vi "Module Not Synced--error.vi"() -> (0 "error out":errorcluster)   [LabVIEW 2020, in "TCP Client.lvlib"]
doc: "Outputs an error cluster containing a custom error code indicating the module events were unable to synchronize.\n_____\nBased on DQMH Project Template 6.0.0.91."
uses:
  TCP Client.lvlib
  <vilib>/Utility/error.llb/Error Cluster From Error Code.vi
  <vilib>/ErrorRing/Error Ring.xnode
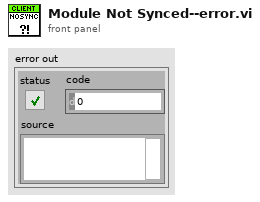
[diagram p1: front panel]
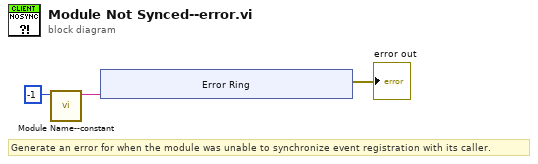
[diagram p0: block diagram]
diagram:
  # "Generate an error for when the module was unable to synchronize event registration with its caller."
  n1 = call "Module Name--constant.vi"("Module ID"=-1) -> ("Module Name"=w2:string)  [unwired: 10 in]
  n2 = xnode "Error Ring"("parameter 0"=w2) -> ("error out"=→"error out":errorcluster)
